vi "Process data.vi"() -> ()   [LabVIEW 2021]
uses:
  <vilib>/Utility/miscctls.llb/LV3DPointTypeDef.ctl
  <vilib>/Platform/TimedLoop/XDataNode/timing_clust.ctl
  <vilib>/Platform/TimedLoop/XDataNode/nitl_modes.ctl
  <vilib>/Platform/TimedLoop/XDataNode/wakeup.ctl
  <vilib>/picture/3D Picture Control/Object/Create Object (drawable).vi
  <vilib>/picture/3D Picture Control/Object/Create Object (name).vi
  <vilib>/picture/3D Picture Control/Object/Add Object (no reference).vi
  Axis Mirorred.vi
  <vilib>/platform/TimedLoop/XDataNode/XDataNode.xnode
  <vilib>/Platform/TimedLoop/XDataNode/XDNodeRunTimeDep.lvlib
  <vilib>/picture/3D Picture Control/NI_3D Picture Control.lvlib
panel:
  in  "Camera Position 2":T1
  in  "eigen assenstelsel 4":dbl[](array[numeric])=[-1.0, 1.0, -1.0]
  in  "Original orient vector 4":dbl[](array[numeric])=[0.0, 0.0, 1.0]
  out "IMU 2":refnum<vi>(3d-picture)
  in  "Enum 4":enum16{"None", "Box", "STL"}(ring)
  in  "Translation 2":cluster{"X":sgl, "Y":sgl, "Z":sgl}
  in  "Color 2":T2={"Red"=1.0, "Green"=0.0, "Blue"=0.0, "Alpha"=1.0}
  in  "Enum 3":enum16{"None", "Box", "STL"}(ring)
  in  "Color":T2={"Red"=1.0, "Green"=0.0, "Blue"=0.0, "Alpha"=1.0}
  in  "Color Rotation":T2={"Red"=1.0, "Green"=0.0, "Blue"=0.0, "Alpha"=1.0}
  in  "Color gravity":T2={"Red"=1.0, "Green"=0.0, "Blue"=0.0, "Alpha"=1.0}
  in  "Up Direction":T1
  in  "Target":T1
  in  "Camera Position":T1
  in  "Translation":cluster{"X":sgl, "Y":sgl, "Z":sgl}
  out "Angle":dbl
  in  "Original orient vector 3":dbl[](array[numeric])=[0.0, 0.0, 1.0]
  in  "eigen assenstelsel 3":dbl[](array[numeric])=[-1.0, 1.0, -1.0]
  in  "Length 2":sgl=2.0 step=0.01
  in  "Enum 2":enum16{"X Axis", "Y Axis", "Z Axis"}(ring)=enum."Z Axis"
  in  "eigen assenstelsel 2":dbl[](array[numeric])=[-1.0, 1.0, -1.0]
  in  "Original orient vector 2":dbl[](array[numeric])=[0.0, 0.0, 1.0]
  out "Rotation vertex":refnum<vi>(3d-picture)
  in  "Length":sgl=2.0 step=0.01
  in  "Enum":enum16{"X Axis", "Y Axis", "Z Axis"}(ring)=enum."Z Axis"
  in  "Original orient vector":dbl[](array[numeric])=[0.0, 0.0, 1.0]
  in  "eigen assenstelsel":dbl[](array[numeric])=[-1.0, 1.0, -1.0]
  out "output variable 4":dbl
  out "output variable 3":dbl
  out "output variable 2":dbl
  out "output variable":dbl
  out "IMU":refnum<vi>(3d-picture)
  in  "stop":bool
  in  "DAQ Port":refnum<visa-resource-name>
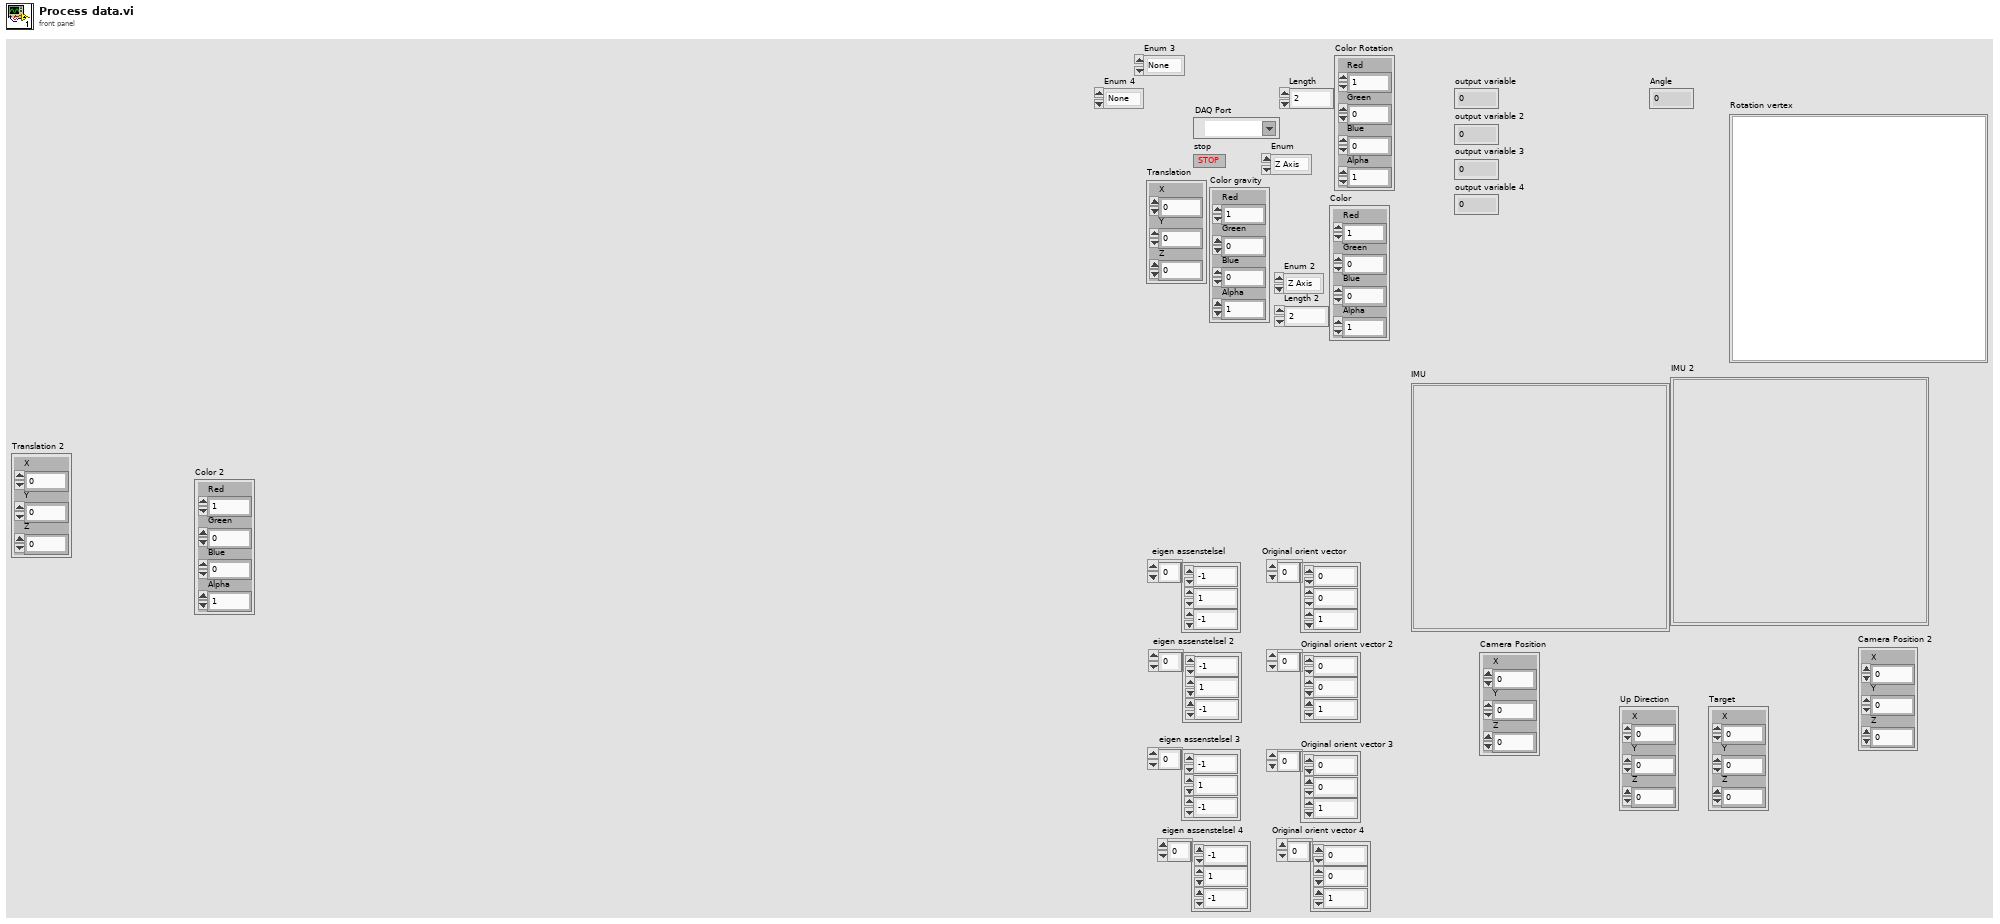
[diagram p1: front panel]
types:
  T1 = typedef "LV3DPointTypeDef.ctl" = cluster{"X":sgl, "Y":sgl, "Z":sgl}
  T2 = cluster{"Red":sgl, "Green":sgl, "Blue":sgl, "Alpha":sgl}
  T3 = typedef "XDNodeRunTimeDep.lvlib/timing_clust.ctl" = cluster{"Expected End [f-1]":u64, "Actual End [f-1]":u64, "Finished Late? [f-1]":bool, "Expected End [i-1]":u64, "Actual End [i-1]":u64, "Finished Late? [i-1]":bool, "Expected Start [i]":u64, "Actual Start [i]":u64, "Expected Start [f]":u64, "Actual Start [f]":u64, "Source Name":string, "Structure Name":string, "Period":i64, "Deadline":i64, "Offset":i64, "Start":i64, "Priority":i32, "Timeout":i32, "Mode":T4, "Wakeup Reason":T5, "Error":errorcluster, "Source Type":string, "Secondary Source Type":string, "Global End Time":u64, "Global Start Time":u64, "Frame Duration":u64, "Iteration Duration":u64, "Assigned CPU":i32, "I/O Scan Engine Mode":u32}
  T4 = typedef "XDNodeRunTimeDep.lvlib/nitl_modes.ctl" = enum32{"No Change", "Process missed periods, maintain original phase", "Discard missed periods, maintain original phase", "Process missed periods, ignore original phase", "Discard missed periods, ignore original phase"}
  T5 = typedef "XDNodeRunTimeDep.lvlib/wakeup.ctl" = enum32{"Normal", "Aborted", "Asynchronous wakeup", "Timing source error", "Timed loop error", "Timeout"}
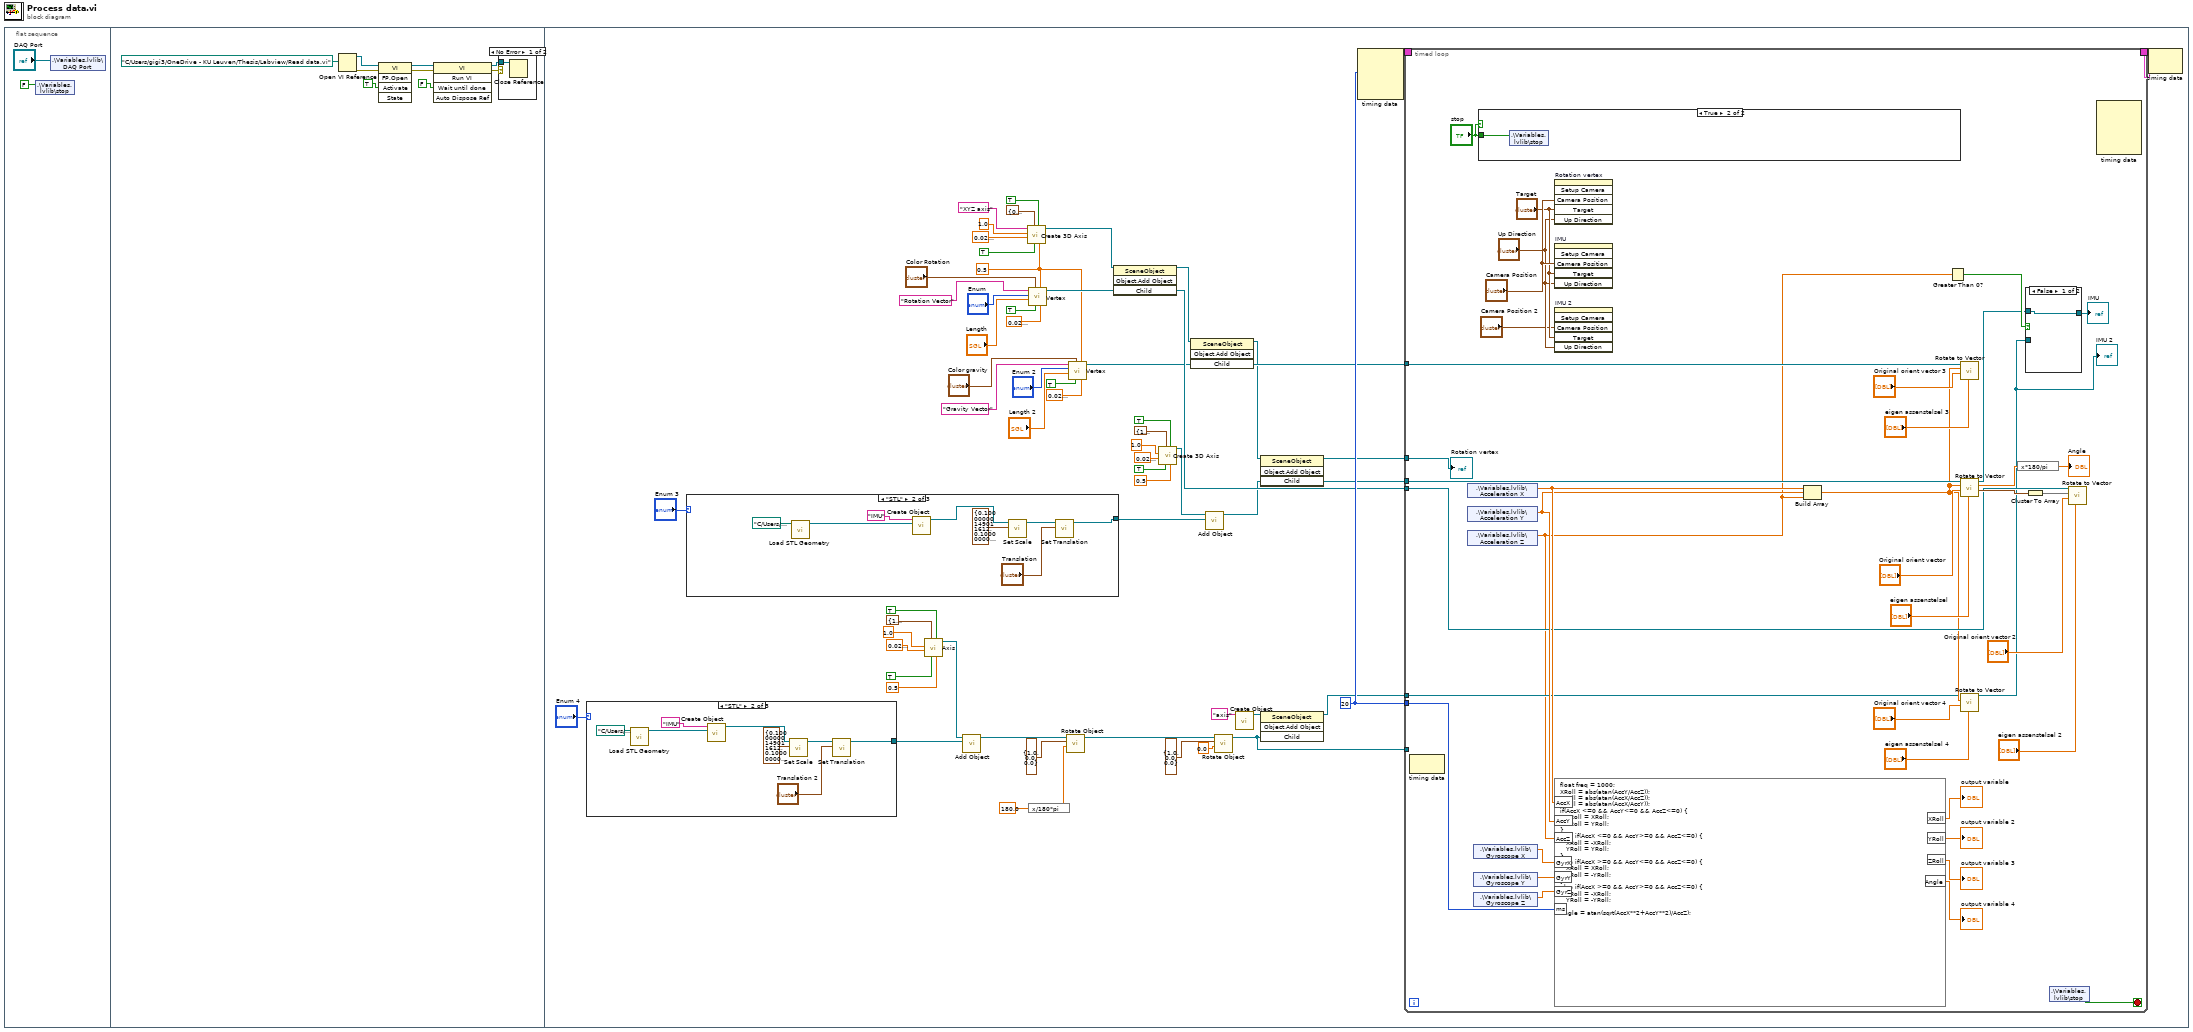
[diagram p0: block diagram]
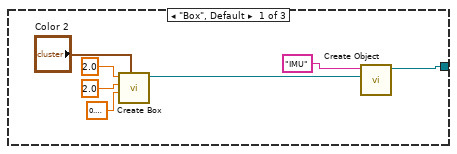
[diagram p3: hidden frame]
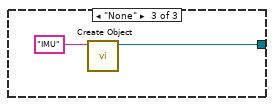
[diagram p4: hidden frame]
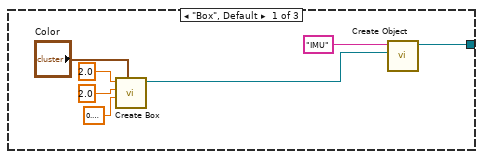
[diagram p5: hidden frame]
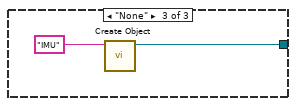
[diagram p6: hidden frame]
diagram:
  n1 = flat-sequence {
    frame #0 {
      n2 = shared-variable ".\\Variables.lvlib\\stop"(FALSE ("stop")) -> ()  [unwired: 1 in, 1 out]
      n3 = shared-variable ".\\Variables.lvlib\\DAQ Port"("DAQ Port") -> ()  [unwired: 1 in, 1 out]
    }
    frame #1 {
      n4 = Open VI Reference(vi path=path "C:/Users/gigi3/OneDrive - KU Leuven/Thesis/Labview/Read data.vi") -> (vi reference=w11:refnum<vi>, error out=w3:errorcluster)  [unwired: 5 in]
      n5 = invoke class="VI" method="FP.Open"(reference=w11, error in=w3, "Activate"=TRUE ("Activate?")) -> (reference out=w10:refnum<vi>, error out=w4:errorcluster)  [unwired: 2 in, 3 out]
      n6 = invoke class="VI" method="Run VI"(reference=w10, error in=w4, "Wait until done"=FALSE ("Wait Until Done")) -> (reference out=w7:refnum<vi>, error out=w5:errorcluster)  [unwired: 2 in, 3 out]
      n7 = case shown="No Error" w5 {
        tunnel: w7 -> [w12 _]
        frame No Error {
          n8 = Close Reference(reference=w12) -> ()  [unwired: 1 in, 1 out]
        }
        frame Error {
        }
      }
    }
    frame #2 {
      w34 = sgl 0.5 ("Character Size")
      w71 = i64 20 ("Period")
      n9 = case shown="\"STL\"" "Enum 4" {
        tunnel: [w75 w81 w89] -> w25
        frame "Box", Default {
          n10 = call <vilib>:"Create Box.vi"("Color"="Color 2", "Length Z"=sgl 0.2, "Length Y"=sgl 2.0, "Length X"=sgl 2.0) -> ("New Box Refnum"=w76:refnum<vi>)  [unwired: 6 in, 1 out]
          n11 = call-poly <vilib>:"Create Object.vi"("Geometry"=w76, "Name"="IMU") -> ("Scene:New Object"=w75:refnum<vi>)  [unwired: 8 in, 1 out]
        }
        frame "STL" {
          n12 = call <vilib>:"Load STL Geometry.vi"("Model File"=path "C:/Users/gigi3/OneDrive - KU Leuven/Thesis/Labview/sparkfun-9dof-imu-breakout-icm-20948-qwiic-1.snapshot.3/SparkFun_IMU_Breakout_ICM-20948 v4 v1.stl") -> ("New Mesh Refnum"=w87:refnum<vi>)  [unwired: 9 in, 1 out]
          n13 = call-poly <vilib>:"Create Object.vi"("Geometry"=w87, "Name"="IMU") -> ("Scene:New Object"=w82:refnum<vi>)  [unwired: 8 in, 1 out]
          n14 = call <vilib>:"Set Scale.vi"("Scale"=cluster{"X":sgl, "Y":sgl, "Z":sgl} {"X"=0.1, "Y"=0.1, "Z"=0.09999999}, "Scene Object"=w82) -> ("Scaled Object"=w84:refnum<vi>)  [unwired: 8 in, 1 out]
          n15 = call <vilib>:"Set Translation.vi"("Translation"="Translation 2", "Scene Object"=w84) -> ("Translated Object"=w81:refnum<vi>)  [unwired: 8 in, 1 out]
        }
        frame "None" {
          n16 = call-poly <vilib>:"Create Object.vi"("Name"="IMU") -> ("Scene:New Object"=w89:refnum<vi>)  [unwired: 9 in, 1 out]
        }
      }
      n17 = case shown="\"STL\"" "Enum 3" {
        tunnel: [w92 w98 w106] -> w35
        frame "Box", Default {
          n18 = call <vilib>:"Create Box.vi"("Color"="Color", "Length Z"=sgl 0.2, "Length Y"=sgl 2.0, "Length X"=sgl 2.0) -> ("New Box Refnum"=w93:refnum<vi>)  [unwired: 6 in, 1 out]
          n19 = call-poly <vilib>:"Create Object.vi"("Geometry"=w93, "Name"="IMU") -> ("Scene:New Object"=w92:refnum<vi>)  [unwired: 8 in, 1 out]
        }
        frame "STL" {
          n20 = call <vilib>:"Load STL Geometry.vi"("Model File"=path "C:/Users/gigi3/OneDrive - KU Leuven/Thesis/Labview/sparkfun-9dof-imu-breakout-icm-20948-qwiic-1.snapshot.3/SparkFun_IMU_Breakout_ICM-20948 v4 v1.stl") -> ("New Mesh Refnum"=w104:refnum<vi>)  [unwired: 9 in, 1 out]
          n21 = call-poly <vilib>:"Create Object.vi"("Geometry"=w104, "Name"="IMU") -> ("Scene:New Object"=w99:refnum<vi>)  [unwired: 8 in, 1 out]
          n22 = call <vilib>:"Set Scale.vi"("Scale"=cluster{"X":sgl, "Y":sgl, "Z":sgl} {"X"=0.1, "Y"=0.1, "Z"=0.09999999}, "Scene Object"=w99) -> ("Scaled Object"=w101:refnum<vi>)  [unwired: 8 in, 1 out]
          n23 = call <vilib>:"Set Translation.vi"("Translation"="Translation", "Scene Object"=w101) -> ("Translated Object"=w98:refnum<vi>)  [unwired: 8 in, 1 out]
        }
        frame "None" {
          n24 = call-poly <vilib>:"Create Object.vi"("Name"="IMU") -> ("Scene:New Object"=w106:refnum<vi>)  [unwired: 9 in, 1 out]
        }
      }
      n25 = call-poly "Axis.vi"("Character Size"=sgl 0.5, "Half plane?"=TRUE, "Axis label?"=TRUE, "Color"=T2 {"Red"=1.0, "Green"=0.0, "Blue"=0.0, "Alpha"=1.0}, "Radius"=sgl 0.03, "Length"=sgl 1.0) -> ("New Object Refnum"=w26:refnum<vi>)  [unwired: 4 in, 1 out]
      n26 = call-poly <vilib>:"Add Object.vi"("New Object In"=w25, "Scene Object In"=w26) -> ("Scene Object Out"=w23:refnum<vi>)  [unwired: 8 in, 1 out]
      n27 = call <vilib>:"Create 3D Axis.vi"("Character Size"=w34, "Half plane?"=TRUE, "Axis label?"=TRUE, "Color"=T2 {"Red"=0.0, "Green"=1.0, "Blue"=0.0, "Alpha"=1.0}, "Radius"=sgl 0.03, "Length"=sgl 1.0, "Name"="XYZ axis") -> ("New Object Refnum"=w54:refnum<vi>)  [unwired: 3 in, 1 out]
      n28 = call "Vertex.vi"("Radius"=sgl 0.03, "Font Size"=w34, "Vertex label?"=TRUE, "Color"="Color Rotation", "Length"="Length", "Enum"="Enum", "Name"="Rotation Vector") -> ("New Object Refnum"=w55:refnum<vi>)  [unwired: 3 in, 1 out]
      n29 = expression code="x/180*pi"(sgl 180.0 ("Angle")) -> (w13:sgl)
      n30 = call <vilib>:"Rotate Object.vi"("Angle"=w13, "Axis"=cluster{"X":sgl, "Y":sgl, "Z":sgl} {"X"=1.0, "Y"=0.0, "Z"=0.0}, "Scene.Object In"=w23) -> ("Scene.Object Out"=w18:refnum<vi>)  [unwired: 7 in, 1 out]
      n31 = call "Vertex.vi"("Radius"=sgl 0.03, "Font Size"=w34, "Vertex label?"=TRUE, "Color"="Color gravity", "Length"="Length 2", "Enum"="Enum 2", "Name"="Gravity Vector") -> ("New Object Refnum"=w47:refnum<vi>)  [unwired: 3 in, 1 out]
      n32 = invoke class="SceneObject" method="Object.Add Object"(reference=w54, "Child"=w55) -> (reference out=w45:refnum<vi>, "Child"=w53:refnum<vi>)  [unwired: 2 in, 2 out]
      n33 = call <vilib>:"Create 3D Axis.vi"("Character Size"=sgl 0.5, "Half plane?"=TRUE, "Axis label?"=TRUE, "Color"=T2 {"Red"=1.0, "Green"=0.0, "Blue"=0.0, "Alpha"=1.0}, "Radius"=sgl 0.03, "Length"=sgl 1.0) -> ("New Object Refnum"=w40:refnum<vi>)  [unwired: 4 in, 1 out]
      n34 = invoke class="SceneObject" method="Object.Add Object"(reference=w45, "Child"=w47) -> (reference out=w44:refnum<vi>, "Child"=w46:refnum<vi>)  [unwired: 2 in, 2 out]
      n35 = call-poly <vilib>:"Add Object.vi"("New Object In"=w35, "Scene Object In"=w40) -> ("Scene Object Out"=w42:refnum<vi>)  [unwired: 8 in, 1 out]
      n36 = call <vilib>:"Rotate Object.vi"("Angle"=sgl 0.0, "Axis"=cluster{"X":sgl, "Y":sgl, "Z":sgl} {"X"=1.0, "Y"=0.0, "Z"=0.0}, "Scene.Object In"=w18) -> ("Scene.Object Out"=w14:refnum<vi>)  [unwired: 7 in, 1 out]
      n37 = call-poly <vilib>:"Create Object.vi"("Name"="axis") -> ("Scene:New Object"=w16:refnum<vi>)  [unwired: 9 in, 1 out]
      n38 = invoke class="SceneObject" method="Object.Add Object"(reference=w44, "Child"=w42) -> (reference out=w43:refnum<vi>, "Child"=w41:refnum<vi>)  [unwired: 2 in, 2 out]
      n39 = invoke class="SceneObject" method="Object.Add Object"(reference=w16, "Child"=w14) -> (reference out=w15:refnum<vi>)  [unwired: 2 in, 3 out]
      n40 = node-c288(w71) -> (w73:T3)  [unwired: 3 in]
      n41 = timed-loop {
        timing: w73 -> [_]
        timing-out: [_] -> w72
        tunnel: w71 -> [w142]
        tunnel: w41 -> [w134]
        tunnel: w53 -> [w129]
        tunnel: w43 -> [w128]
        tunnel: w46 -> [w127]
        tunnel: w15 -> [w113]
        tunnel: w14 -> [_]
        stop <- w135 stop-if-true
        n42 = node-c288() -> ()  [unwired: 1 in, 1 out]
        n43 = shared-variable ".\\Variables.lvlib\\Acceleration X"() -> (w141:dbl)  [unwired: 1 in, 1 out]
        n44 = shared-variable ".\\Variables.lvlib\\Acceleration Y"() -> (w140:dbl)  [unwired: 1 in, 1 out]
        n45 = shared-variable ".\\Variables.lvlib\\Acceleration Z"() -> (w112:dbl)  [unwired: 1 in, 1 out]
        n46 = shared-variable ".\\Variables.lvlib\\Gyroscope X"() -> (w145:dbl)  [unwired: 1 in, 1 out]
        n47 = shared-variable ".\\Variables.lvlib\\Gyroscope Y"() -> (w144:dbl)  [unwired: 1 in, 1 out]
        n48 = shared-variable ".\\Variables.lvlib\\Gyroscope Z"() -> (w143:dbl)  [unwired: 1 in, 1 out]
        n49 = case shown="True" "stop" {
          tunnel: "stop" -> [_ w151]
          frame False {
          }
          frame True {
            n50 = shared-variable ".\\Variables.lvlib\\stop"(w151) -> ()  [unwired: 1 in, 1 out]
          }
        }
        n51 = invoke on="Rotation vertex" class="SceneGraphDisp (strict)" method="Setup Camera"("Camera Position"="Camera Position", "Target"="Target", "Up Direction"="Up Direction") -> ()  [unwired: 3 in, 6 out]
        n52 = invoke on="IMU" class="SceneGraphDisp (strict)" method="Setup Camera"("Camera Position"="Camera Position", "Target"="Target", "Up Direction"="Up Direction") -> ()  [unwired: 3 in, 6 out]
        n53 = invoke on="IMU 2" class="SceneGraphDisp (strict)" method="Setup Camera"("Camera Position"="Camera Position 2", "Target"="Target", "Up Direction"="Up Direction") -> ()  [unwired: 3 in, 6 out]
        n54 = formula code="float freq = 1000;\nXRoll = abs(atan(AccY/AccZ));\nYRoll = abs(atan(AccX/AccZ));\nZRoll = abs(atan(AccX/AccY));\nif(AccX <=0 && AccY<=0 && AccZ<=0) {\n   XRoll = XRoll;\n   YRoll = YRoll;\n}\nelse if(AccX <=0 && AccY>=0 && AccZ<=0) {\n   XRoll = -XRoll;\n   YRoll = YRoll;\n}\nelse if(AccX >=0 && AccY<=0 && AccZ<=0) {\n   XRoll = XRoll;\n   YRoll = -YRoll;\n}\nelse if(AccX >=0 && AccY>=0 && AccZ<=0) {\n   XRoll = -XRoll;\n   YRoll = -YRoll;\n}\nAngle = atan(sqrt(AccX**2+AccY**2)/AccZ);"("AccX"=w141, "AccY"=w140, "AccZ"=w112, "GyrX"=w145, "GyrY"=w144, "GyrZ"=w143, "ms"=w142) -> ("XRoll"=→"output variable":dbl, "YRoll"=→"output variable 2":dbl, "ZRoll"=→"output variable 3":dbl, "Angle"=→"output variable 4":dbl)
        n55 = Build Array(w141, w140, w112) -> (w120:dbl[])
        n56 = Greater Than 0?(x=w112) -> (x > 0?=w111:bool)
        n57 = call "Rotate to Vector.vi"("eigen assenstelsel"="eigen assenstelsel 3", "Original orient vector"="Original orient vector 3", "input vector"=w120, "Scene Object"=w127) -> ()  [unwired: 4 in, 4 out]
        n58 = call "Rotate to Vector.vi"("eigen assenstelsel"="eigen assenstelsel", "Original orient vector"="Original orient vector", "input vector"=w120, "Scene Object"=w134) -> ("Axis"=w131:cluster{"X":sgl, "Y":sgl, "Z":sgl}, "arccos(x)"=w122:dbl, "Rotated Scene Object"=w110:refnum<vi>)  [unwired: 4 in, 1 out]
        n59 = call "Rotate to Vector.vi"("eigen assenstelsel"="eigen assenstelsel 4", "Original orient vector"="Original orient vector 4", "input vector"=w120, "Scene Object"=w113) -> ("Rotated Scene Object"=w108:refnum<vi>)  [unwired: 4 in, 3 out]
        "IMU 2" <- w108
        n60 = expression code="x*180/pi"(w122) -> (→"Angle":dbl)
        n61 = case shown="False" w111 {
          tunnel: w108 -> [_ w148]
          tunnel: w110 -> [w147 _]
          tunnel: [w147 w148] -> w109
          frame False {
          }
          frame True {
          }
        }
        "IMU" <- w109
        n62 = Cluster To Array(cluster=w131) -> (array=w130:sgl[])
        n63 = shared-variable ".\\Variables.lvlib\\stop"() -> (w135:bool)  [unwired: 1 in, 1 out]
        n64 = call "Rotate to Vector.vi"("eigen assenstelsel"="eigen assenstelsel 2", "Original orient vector"="Original orient vector 2", "input vector"=w130, "Scene Object"=w129) -> ()  [unwired: 4 in, 4 out]
        n65 = node-c288() -> ()  [unwired: 5 in, 1 out]
        "Rotation vertex" <- w128
      }
      n66 = node-c288(w72) -> ()  [unwired: 1 out]
    }
  }
